vi "Control Aero Overhead Strut.vi"() -> ()   [LabVIEW 2022 SP3]
panel:
  in  "Desired Increment (mm)":dbl
  out "Start Position":dbl
  out "End Position":dbl
  out "Increment":dbl
  in  "Down Calibration ms/mm":dbl=50.1
  in  "Up Calibration ms/mm":dbl=62.0
  out "Actual Run Period (ms)":u32
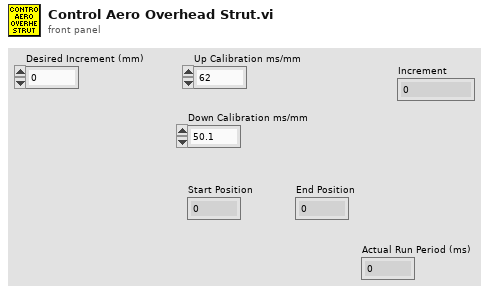
[diagram p1: front panel]
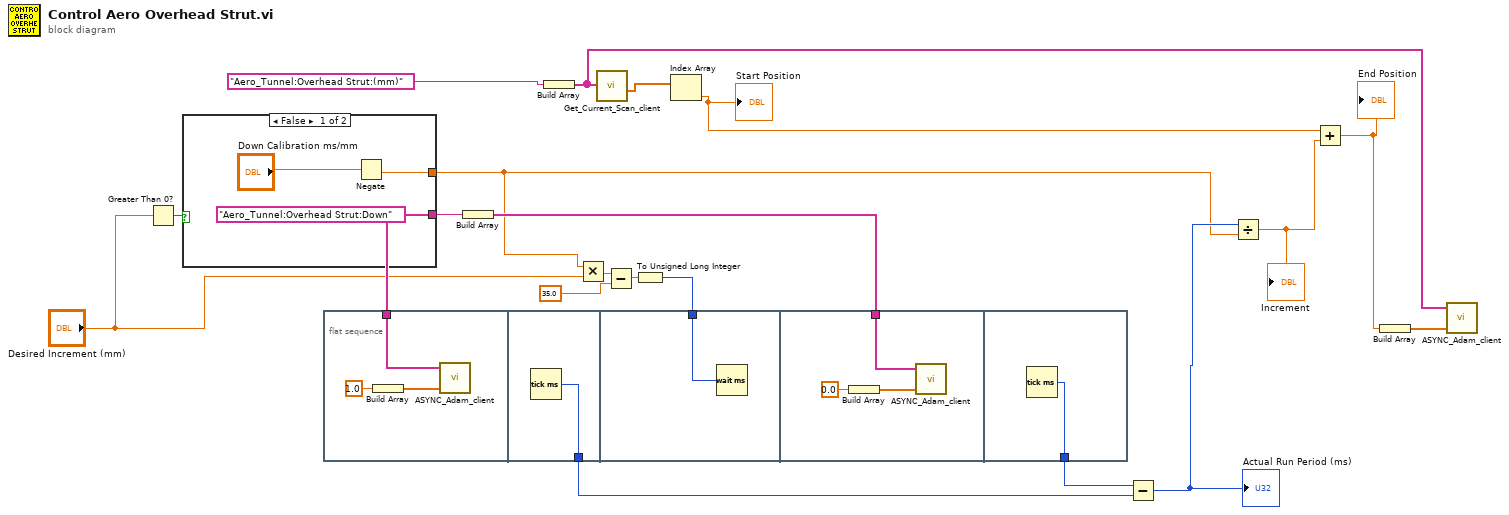
[diagram p0: block diagram]
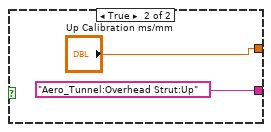
[diagram p2: hidden frame]
diagram:
  n1 = Greater Than 0?(x="Desired Increment (mm)") -> (x > 0?=w6:bool)
  n2 = case shown="False" w6 {
    tunnel: ["Aero_Tunnel:Overhead Strut:Down" "Aero_Tunnel:Overhead Strut:Up"] -> w19
    tunnel: [w20 "Up Calibration ms/mm"] -> w2
    frame False {
      n3 = Negate(x="Down Calibration ms/mm") -> (-x=w20:dbl)
    }
    frame True {
    }
  }
  n4 = flat-sequence {
    tunnel: w18 -> [w26]
    tunnel: [w28] -> w17
    tunnel: w1 -> [w29]
    tunnel: w18 -> [w30]
    tunnel: [w33] -> w16
    frame #0 {
      n5 = Build Array(1.0) -> (w27:dbl[])
      n6 = call "ASYNC_Adam_client.vi"("Values"=w27, "Channel Names"=w26) -> ()  [unwired: 1 in, 2 out]
    }
    frame #1 {
      n7 = Tick Count (ms)() -> (millisecond timer value=w28:u32)
    }
    frame #2 {
      n8 = Wait (ms)(milliseconds to wait=w29) -> ()  [unwired: 1 out]
    }
    frame #3 {
      n9 = Build Array(0.0) -> (w31:dbl[])
      n10 = call "ASYNC_Adam_client.vi"("Values"=w31, "Channel Names"=w30) -> ()  [unwired: 1 in, 2 out]
    }
    frame #4 {
      n11 = Tick Count (ms)() -> (millisecond timer value=w33:u32)
    }
  }
  n12 = Build Array(w19) -> (w18:string[])
  n13 = Build Array("Aero_Tunnel:Overhead Strut:(mm)") -> (w8:string[])
  n14 = Multiply(x=w2, y="Desired Increment (mm)") -> (x*y=w4:dbl)
  n15 = call "Get_Current_Scan_client.vi"("multipleChannels"=w8) -> ("Numerical Values"=w14:dbl[])  [unwired: 1 in, 3 out]
  n16 = Subtract(x=w4, y=35.0) -> (x-y=w3:dbl)
  n17 = To Unsigned Long Integer(number=w3) -> (unsigned 32bit integer=w1:u32)
  n18 = Index Array(array=w14) -> (element=w12:dbl)  [unwired: 1 in]
  "Start Position" <- w12
  n19 = Subtract(x=w16, y=w17) -> (x-y=w13:u32)
  "Actual Run Period (ms)" <- w13
  n20 = Divide(x=w13, y=w2) -> (x/y=w11:dbl)
  "Increment" <- w11
  n21 = Add(x=w12, y=w11) -> (x+y=w9:dbl)
  "End Position" <- w9
  n22 = Build Array(w9) -> (w10:dbl[])
  n23 = call "ASYNC_Adam_client.vi"("Values"=w10, "Channel Names"=w8) -> ()  [unwired: 1 in, 2 out]
